vi "Interface Read select.vi"(8 "error in (no error)":errorcluster, 9 "timeout":i32=10000, 10 "bytes to read":i32, 11 "TCP interface in":refnum<class "TCP Interface.lvclass">) -> (0 "error out":errorcluster, 1 "timed out?":bool, 2 "data":string, 3 "TCP interface out":refnum<class "TCP Interface.lvclass">)   [LabVIEW 2021, in "TCP Interface.lvclass"]
doc: "Reads from the established TCP connection stored in the class."
uses:
  TCP Interface.lvclass
  TCP Interface.lvclass/TCP Interface.ctl
  <vilib>/Utility/error.llb/Clear Errors.vi
  TCP Shared Components/TCP Shared Components.lvlib
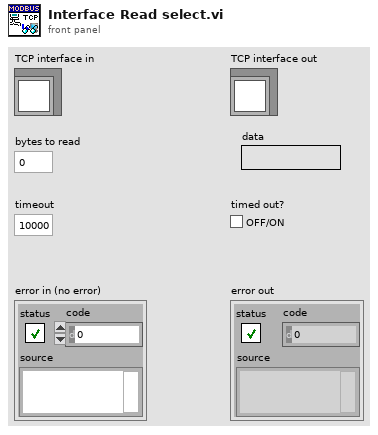
[diagram p1: front panel]
types:
  T1 = enum16{"Standard", "Buffered", "CRLF", "Immediate"}
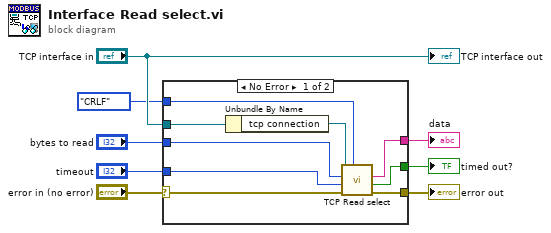
[diagram p0: block diagram]
diagram:
  n1 = case shown="No Error" "error in (no error)" {
    selector: "error in (no error)" -> [w13 w18]
    tunnel: "TCP interface in" -> [w17 _]
    tunnel: "bytes to read" -> [w16 _]
    tunnel: "timeout" -> [w14 _]
    tunnel: [w12 w18] -> w5
    tunnel: [w11 _] -> w4
    tunnel: [w10 _] -> w2
    tunnel: T1."CRLF" ("mode (standard)") -> [w9 _]
    frame No Error {
      n2 = Unbundle By Name(w17) -> ("tcp connection"=w15:refnum<k5>)
      n3 = call "TCP Read select.vi"("mode (standard)"=w9, "error in (no error)"=w13, "timeout"=w14, "bytes to read"=w16, "connection ID"=w15) -> ("error out"=w12:errorcluster, "timed out?"=w11:bool, "data"=w10:string)  [unwired: 4 in]
    }
    frame Error {
    }
  }
  "error out" <- w5
  "timed out?" <- w4
  "data" <- w2
  "TCP interface out" <- "TCP interface in"
